vi "Launch Process.vi"(8 "error in (no error)":errorcluster, 11 "Process in":refnum<class "Process.lvclass">) -> (0 "error out":errorcluster, 3 "Process out":refnum<class "Process.lvclass">)   [LabVIEW 2020, in "Process.lvclass"]
doc: "This VI launches the process vi. The algorithm is optimized using the same tricks as Actor Framework."
uses:
  Process.lvclass
  <vilib>/Utility/error.llb/Error Cluster From Error Code.vi
  <vilib>/ErrorRing/Error Ring.xnode
  Process.lvclass/Process.ctl
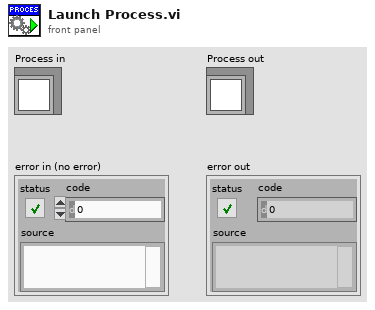
[diagram p1: front panel]
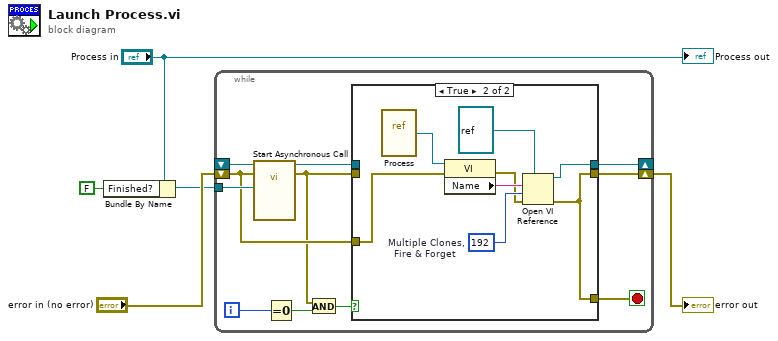
[diagram p0: block diagram]
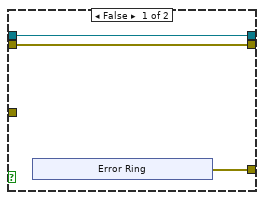
[diagram p2: hidden frame]
diagram:
  n1 = Bundle By Name(cluster="Process in", "Finished?"=FALSE) -> (w2:refnum<class "Process.lvclass">)
  n2 = while {
    tunnel: w2 -> [w16]
    shift-right: [w7] -> w4
    shift-left: "error in (no error)" -> [w8]
    shift-right: [w12] -> _
    shift-left: _ -> [w15]
    i -> [w14]
    stop <- w9 stop-if-true
    n3 = call-by-ref "Start Asynchronous Call"(reference=w15, error in=w8, "Process In"=w16) -> (reference out=w11:refnum<vi>, error out=w6:errorcluster)  [unwired: 11 in]
    n4 = Equal To 0?(x=w14) -> (x = 0?=w13:bool)
    n5 = And(x=w6, y=w13) -> (x .and. y?=w10:bool)
    n6 = case shown="True" w10 {
      tunnel: [w19 w26] -> w12
      tunnel: w11 -> [w19 _]
      tunnel: [w18 w24] -> w9
      tunnel: w8 -> [_ w25]
      tunnel: [w17 w24] -> w7
      tunnel: w6 -> [w17 _]
      frame False {
        n7 = xnode "Error Ring"() -> ("error out"=w18:errorcluster)
      }
      frame True {
        w28 = 192  # Multiple Clones,   Fire & Forget
        n8 = vi-ref "Process.vi"() -> (w30:refnum<vi>)
        n9 = property class="VI"(reference=w30, error in=w25) -> (error out=w27:errorcluster, "Name"=w31:string)  [unwired: 1 out]
        n10 = Open VI Reference(type specifier VI Refnum (for type only)=refnum<vi> refnum, vi path=w31, options=w28, error in (no error)=w27) -> (vi reference=w26:refnum<vi>, error out=w24:errorcluster)  [unwired: 2 in]
      }
    }
  }
  "error out" <- w4
  "Process out" <- "Process in"
